vi "Acquire waveforms.vi"(8 "Error In":errorcluster, 9 "Channel String":string="0,1", 11 "Oscilloscope Board Name":refnum<k15>) -> (0 "Error Out":errorcluster, 1 "Acquisition Result":T1={"Traces"=[], "Relative t0 [s]"=1000.0, "Sample Rate [1/s]"=1000.0, "No. of points"=0, "Absolute t0 [s]"=1000.0, "dT [s]"=1000.0, "Update rate [1/s]"=0.0, "Auto Triggered"=FALSE, "Stop"=FALSE} {"Update rate [1/s]" format="%_3p"}, 2 "Waveforms Out":waveform(dbl)[](graph), 3 "Oscilloscope Board Name Out":refnum<k15>, 5 "wfm info":T2(array[cluster]) {"reserved2" format="%.2f"; "reserved1" format="%.2f"; "offset" format="%^.3e"; "gain" format="%^.3e"; "xIncrement" format="%^.3e"; "relativeInitialX" format="%^.3e"; "absoluteInitialX" format="%^.3e"})   [LabVIEW 2019]
uses:
  Controls/Acquisition Result.ctl
  <instrlib>/niScope/Controls/niScope timestamp type.ctl
  <instrlib>/niScope/Acquire/Fetch/niScope Multi Fetch WDT.vi
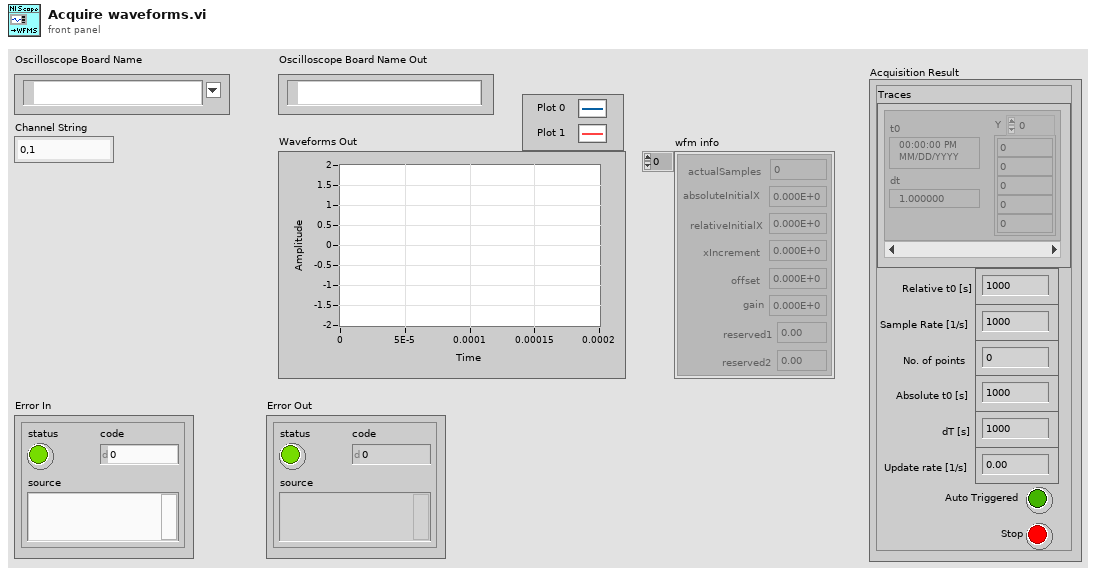
[diagram p1: front panel]
types:
  T1 = typedef "Acquisition Result.ctl" = cluster{"Traces":waveform(sgl)[], "Relative t0 [s]":dbl, "Sample Rate [1/s]":dbl, "No. of points":i32, "Absolute t0 [s]":dbl, "dT [s]":dbl, "Update rate [1/s]":dbl, "Auto Triggered":bool, "Stop":bool}
  T2 = cluster{"actualSamples":i32, "absoluteInitialX":dbl, "relativeInitialX":dbl, "xIncrement":dbl, "offset":dbl, "gain":dbl, "reserved1":dbl, "reserved2":dbl}[]
  T3 = typedef "niScope timestamp type.ctl" = i32
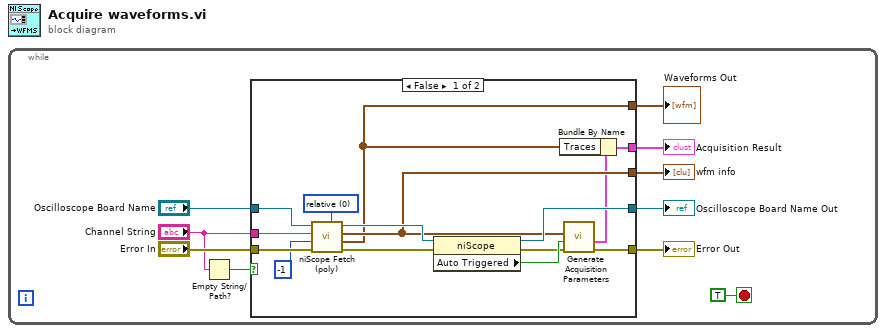
[diagram p0: block diagram]
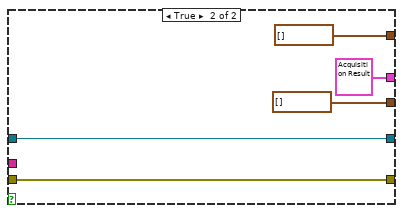
[diagram p2: hidden frame]
diagram:
  n1 = while {
    stop <- TRUE stop-if-true
    n2 = Empty String/Path?(string/path="Channel String") -> (empty?=w10:bool)
    n3 = case shown="False" w10 {
      tunnel: "Oscilloscope Board Name" -> [w25 w29]
      tunnel: "Error In" -> [w24 w30]
      tunnel: "Channel String" -> [w23 _]
      tunnel: [w14 w30] -> w6
      tunnel: [w19 w29] -> w7
      tunnel: [w12 waveform(dbl)[] [] ("wfm")] -> w8
      tunnel: [w17 T2 [] ("wfm info")] -> w4
      tunnel: [w11 T1 {"Traces"=[], "Relative t0 [s]"=1000.0, "Sample Rate [1/s]"=1000.0, "No. of points"=0, "Absolute t0 [s]"=1000.0, "dT [s]"=1000.0, "Update rate [1/s]"=0.0, "Auto Triggered"=FALSE, "Stop"=FALSE} ("Acquisition Result")] -> w1
      frame False {
        w22 = T3 0 items=["relative", "absolute"] ("timestamp Type")
        n4 = call-poly <instrlib>:"niScope Fetch (poly).vi"("timestamp Type"=w22, "error in"=w24, "numSamples"=-1, "channels"=w23, "instrument handle"=w25) -> ("error out"=w18:errorcluster, "wfm"=w12:waveform(dbl)[], "wfm info"=w17:T2, "instrument handle out"=w20:refnum<k15>)  [unwired: 3 in]
        n5 = property class="niScope"(reference=w20, error in=w18) -> (reference out=w19:refnum<k15>, error out=w15:errorcluster, "Auto Triggered"=w16:bool)
        n6 = call "Generate Acquisition Parameters.vi"("Error In"=w15, "Auto Triggered?"=w16, "wfm info"=w17) -> ("Error Out"=w14:errorcluster, "Acquisition Result"=w13:T1)  [unwired: 7 in]
        n7 = Bundle By Name(cluster=w13, "Traces"=w12) -> (w11:T1)
      }
      frame True {
      }
    }
    "Waveforms Out" <- w8
    "wfm info" <- w4
    "Acquisition Result" <- w1
    "Oscilloscope Board Name Out" <- w7
    "Error Out" <- w6
  }
